vi "Triggered Measure.vi"(6 "Restore Range if Checked?(T)":bool=TRUE, 7 "Check Range?(T)":bool=TRUE, 8 "error in (no error)":errorcluster, 9 "Max Time (-1ms)":i32=-1, 10 "Measurements to Acquire(1)":i32=1 min=0, 11 "DMM Driver in":refnum<class "DMM Driver.lvclass">) -> (0 "error out":errorcluster, 1 "Function":T2, 2 "Measurements":dbl[](array[numeric]), 3 "DMM Driver out":refnum<class "DMM Driver.lvclass">, 4 "Range":dbl, 5 "Digit Resolution(5½)":T1=enum."5½")   [LabVIEW 2020, in "DMM.lvlib" / "DMM Driver.lvclass"]
doc: "Perform a triggered measurement operation on the DMM. The trigger options are specified using 'Configure Trigger'.\nThe measurements are returned together with the current configuration of the DMM.\nIf requested the DMM will autorange before performing the measurements. The DMM range can be restored after the measurements."
uses:
  DMM Driver.lvclass
  Controls/Ctl_DigitResolution.ctl
  DMM.lvlib
  Controls/Ctl_Function.ctl
  Controls/Community/Ctl_Config.ctl
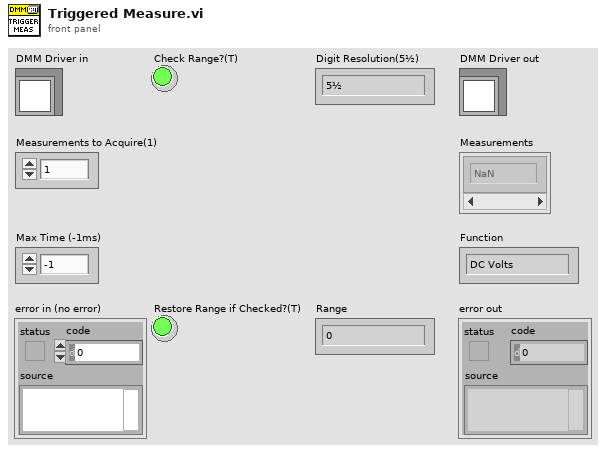
[diagram p1: front panel]
types:
  T1 = typedef "DMM.lvlib/Ctl_DigitResolution.ctl" = enum8{"3½", "4½", "5½", "6½", "7½"}
  T2 = typedef "DMM.lvlib/Ctl_Function.ctl" = enum8{"DC Volts", "AC Volts", "DC Current", "AC Current", "2-wire Resistance", "4-wire Resistance", "Diode", "Frequency", "Period", "AC Volts DC Coupled", "Capacitance", "Inductance", "Temperature"}
  T3 = typedef "DMM.lvlib/Ctl_Config.ctl" = cluster{"Function":T2, "Range":dbl, "Digit Resolution(5½)":T1}
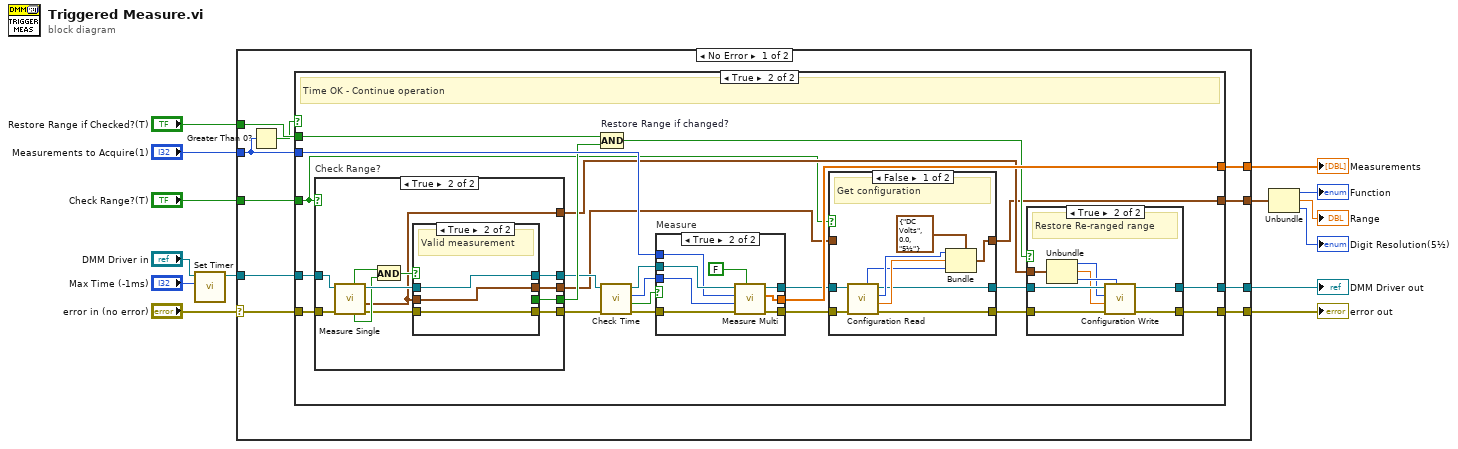
[diagram p0: block diagram]
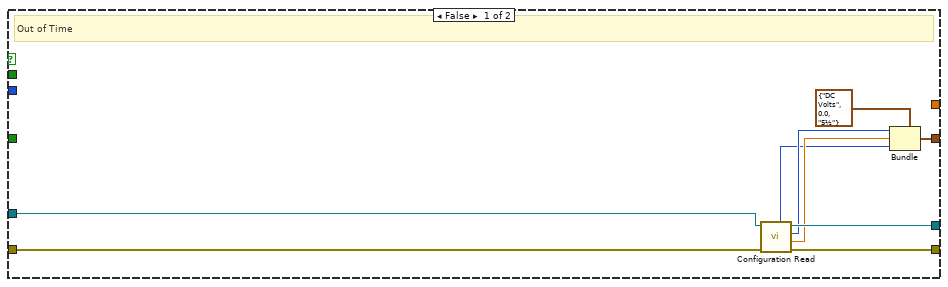
[diagram p2: hidden frame]
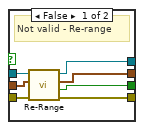
[diagram p7: hidden frame]
diagram:
  n1 = call "Set Timer.vi"("Max Time (-1ms)"="Max Time (-1ms)", "DMM Driver in"="DMM Driver in") -> ("DMM Driver out"=w10:refnum<class "DMM Driver.lvclass">)  [unwired: 9 in]
  n2 = case shown="No Error" "error in (no error)" {
    selector: "error in (no error)" -> [w23 w114]
    tunnel: [w19 w114] -> w13
    tunnel: [w22 w113] -> w11
    tunnel: w10 -> [w24 w113]
    tunnel: "Measurements to Acquire(1)" -> [w21 _]
    tunnel: [w20 _] -> w6
    tunnel: [w18 _] -> w7
    tunnel: "Restore Range if Checked?(T)" -> [w17 _]
    tunnel: "Check Range?(T)" -> [w15 _]
    frame No Error {
      n3 = Greater Than 0?(x=w21) -> (x > 0?=w16:bool)
      n4 = case shown="True" w16 {
        tunnel: w24 -> [w33 w51]
        tunnel: w23 -> [w31 w50]
        tunnel: [w30 w56] -> w19
        tunnel: [w32 w55] -> w22
        tunnel: w21 -> [_ w54]
        tunnel: [_ w53] -> w20
        tunnel: [w26 w35] -> w18
        tunnel: w17 -> [_ w52]
        tunnel: w15 -> [_ w40]
        frame False {
          # "Out of Time"
          n5 = call-dynamic "Configuration Read.vi"("error in (no error)"=w31, "DMM Driver in"=w33) -> ("error out"=w30:errorcluster, "Range"=w29:dbl, "Function"=w28:T2, "DMM Driver out"=w32:refnum<class "DMM Driver.lvclass">, "Digit Resolution(5½)"=w27:T1)  [unwired: 5 in]
          n6 = Bundle(cluster=T3 {"Function"=enum."DC Volts", "Range"=0.0, "Digit Resolution(5½)"=enum."5½"} ("Config"), "Function"=w28, "Range"=w29, "Digit Resolution(5½)"=w27) -> (w26:T3)
        }
        frame True {
          # "Time OK - Continue operation"
          n7 = case "Check Range?" shown="True" w40 {
            tunnel: w51 -> [w90 w102]
            tunnel: [w90 w99] -> w43
            tunnel: w50 -> [w89 w101]
            tunnel: [w89 w94] -> w42
            tunnel: [_ w93] -> w49
            tunnel: [_ w92] -> w41
            tunnel: [_ w91] -> w34
            frame False {
            }
            frame True {
              n8 = call "Measure Single.vi"("error in (no error)"=w101, "DMM Driver in"=w102) -> ("error out"=w95:errorcluster, "Config"=w92:T3, "DMM Driver out"=w100:refnum<class "DMM Driver.lvclass">, "Valid measurement?"=w97:bool, "Finished?"=w98:bool)  [unwired: 4 in, 1 out]
              n9 = And(x=w98, y=w97) -> (x .and. y?=w96:bool)
              n10 = case shown="True" w96 {
                tunnel: [w109 w110] -> w94
                tunnel: w95 -> [w106 w110]
                tunnel: [w108 w112] -> w99
                tunnel: w100 -> [w107 w112]
                tunnel: [w104 w111] -> w91
                tunnel: w92 -> [w105 w111]
                tunnel: [w103 _] -> w93
                frame False {
                  # "Not valid - Re-range"
                  n11 = call "Re-Range.vi"("error in (no error)"=w106, "Config in"=w105, "DMM Driver in"=w107) -> ("error out"=w109:errorcluster, "Success?"=w103:bool, "Config out"=w104:T3, "DMM Driver out"=w108:refnum<class "DMM Driver.lvclass">)  [unwired: 5 in]
                }
                frame True {
                  # "Valid measurement"
                }
              }
            }
          }
          n12 = Compound Arithmetic op=AND "Restore Range if changed?"(w52, w49) -> (w45:bool)
          n13 = call "Check Time.vi"("error in (no error)"=w42, "DMM Driver in"=w43) -> ("error out"=w48:errorcluster, "Time OK?"=w44:bool, "Remaining Time"=w46:i32, "DMM Driver out"=w47:refnum<class "DMM Driver.lvclass">)  [unwired: 6 in]
          n14 = case "Measure" shown="True" w44 {
            tunnel: w48 -> [w69 w78]
            tunnel: w47 -> [w70 w77]
            tunnel: w46 -> [_ w76]
            tunnel: [w69 w75] -> w36
            tunnel: [w70 w74] -> w38
            tunnel: [_ w73] -> w53
            tunnel: w54 -> [_ w72]
            frame False {
            }
            frame True {
              n15 = call-dynamic "Measure Multi.vi"("Config for Immediate Measure?(T)"=FALSE, "error in (no error)"=w78, "Max Time (-1ms)"=w76, "Measurements to Acquire(1)"=w72, "DMM Driver in"=w77) -> ("error out"=w75:errorcluster, "Measurements"=w73:dbl[], "DMM Driver out"=w74:refnum<class "DMM Driver.lvclass">)  [unwired: 4 in]
            }
          }
          n16 = case shown="False" w40 {
            tunnel: [w59 w68] -> w39
            tunnel: w38 -> [w61 w68]
            tunnel: [w57 w67] -> w37
            tunnel: w36 -> [w58 w67]
            tunnel: [w60 w66] -> w35
            tunnel: w34 -> [_ w66]
            frame False {
              # "Get configuration"
              n17 = call-dynamic "Configuration Read.vi"("error in (no error)"=w58, "DMM Driver in"=w61) -> ("error out"=w57:errorcluster, "Range"=w65:dbl, "Function"=w64:T2, "DMM Driver out"=w59:refnum<class "DMM Driver.lvclass">, "Digit Resolution(5½)"=w63:T1)  [unwired: 5 in]
              n18 = Bundle(cluster=T3 {"Function"=enum."DC Volts", "Range"=0.0, "Digit Resolution(5½)"=enum."5½"} ("Config"), "Function"=w64, "Range"=w65, "Digit Resolution(5½)"=w63) -> (w60:T3)
            }
            frame True {
              # "Config known - Skip"
            }
          }
          n19 = case "Restore Range if changed?" shown="True" w45 {
            tunnel: [w80 w81] -> w56
            tunnel: w37 -> [w80 w82]
            tunnel: [w79 w86] -> w55
            tunnel: w39 -> [w79 w87]
            tunnel: w41 -> [_ w88]
            frame False {
            }
            frame True {
              # "Restore Re-ranged range"
              n20 = Unbundle(w88) -> ("Function"=w84:T2, "Range"=w83:dbl, "Digit Resolution(5½)"=w85:T1)
              n21 = call "Configuration Write.vi"("Digit Resolution(5½)"=w85, "error in (no error)"=w82, "Range"=w83, "Function"=w84, "DMM Driver in"=w87) -> ("error out"=w81:errorcluster, "DMM Driver out"=w86:refnum<class "DMM Driver.lvclass">)  [unwired: 4 in, 1 out]
            }
          }
        }
      }
    }
    frame Error {
    }
  }
  "error out" <- w13
  "DMM Driver out" <- w11
  "Measurements" <- w6
  n22 = Unbundle(w7) -> ("Function"=→"Function":T2, "Range"=→"Range":dbl, "Digit Resolution(5½)"=→"Digit Resolution(5½)":T1)
